vi "Logger Server.vi"(11 "error in (no error)":errorcluster) -> (15 "error out":errorcluster)   [LabVIEW 2018]
uses:
  Logger Global.vi
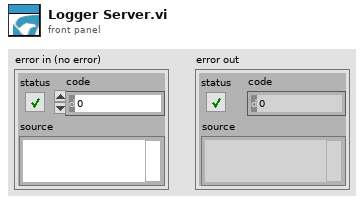
[diagram p1: front panel]
types:
  T1 = cluster{"Log File Input":string, "Log Entry Type":enum16{"STANDARD", "WARNING", "CRITICAL"}}
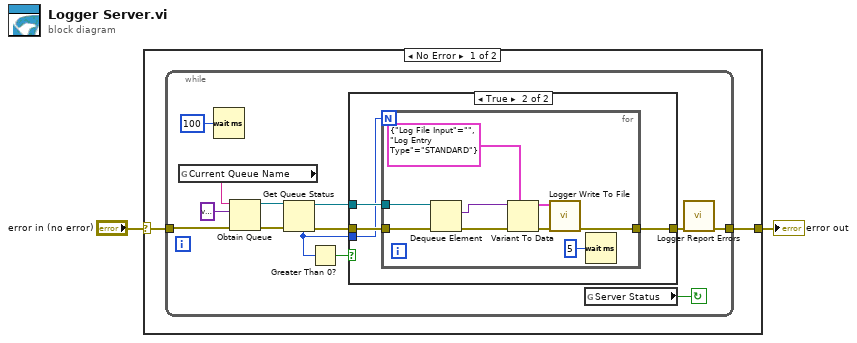
[diagram p0: block diagram]
diagram:
  n1 = case shown="No Error" "error in (no error)" {
    selector: "error in (no error)" -> [w4 w32]
    tunnel: [w3 w32] -> w1
    frame No Error {
      n2 = while {
        tunnel: w4 -> [w9]
        tunnel: [w5] -> w3
        stop <- w12 continue-if-true
        n3 = global read "Logger Global.vi" "Current Queue Name"() -> (w7:string)
        n4 = Wait (ms)(milliseconds to wait=u32 100) -> ()  [unwired: 1 out]
        n5 = Obtain Queue(name (unnamed)=w7, element data type=variant, error in (no error)=w9) -> (queue out=w8:refnum<queue>, error out=w10:errorcluster)  [unwired: 2 in, 1 out]
        n6 = Get Queue Status(queue=w8, error in (no error)=w10) -> (queue out=w15:refnum<queue>, error out=w16:errorcluster, # elements in queue=w13:i32)  [unwired: 1 in, 5 out]
        n7 = Greater Than 0?(x=w13) -> (x > 0?=w14:bool)
        n8 = case shown="True" w14 {
          tunnel: w16 -> [w18 w22]
          tunnel: w15 -> [_ w21]
          tunnel: w13 -> [_ w20]
          tunnel: [w18 w19] -> w11
          frame False {
          }
          frame True {
            n9 = for {
              N: w20 -> [_]
              tunnel: w22 -> [w31]
              tunnel: w21 -> [w30]
              tunnel: [w26] -> w19
              n10 = Dequeue Element(queue=w30, error in (no error)=w31) -> (element=w28:variant, error out=w29:errorcluster)  [unwired: 1 in, 2 out]
              n11 = Variant To Data(error in=w29, type=T1 {"Log File Input"="", "Log Entry Type"=enum."STANDARD"} ("Log File Input"), Variant=w28) -> (data=w23:T1, error out=w27:errorcluster)
              n12 = call "Logger Write To File.vi"("Log File Input"=w23, "error in (no error)"=w27) -> ("error out"=w26:errorcluster)  [unwired: 13 in]
              n13 = Wait (ms)(milliseconds to wait=u32 5) -> ()  [unwired: 1 out]
            }
          }
        }
        n14 = global read "Logger Global.vi" "Server Status"() -> (w12:bool)
        n15 = call "Logger Report Errors.vi"("error in (no error)"=w11) -> ("error out"=w5:errorcluster)  [unwired: 14 in]
      }
    }
    frame Error {
    }
  }
  "error out" <- w1
